vi "PID.vi"(7 "KD":dbl, 8 "Initial feedback in":dbl, 9 "KI":dbl, 10 "Error in":dbl, 11 "KP":dbl) -> (3 "PIDout":dbl)   [LabVIEW 2016]
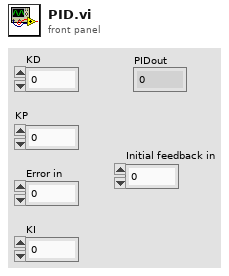
[diagram p1: front panel]
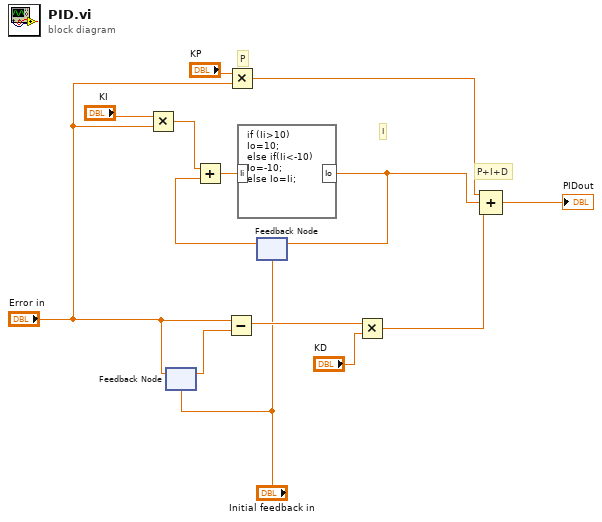
[diagram p0: block diagram]
diagram:
  # "P+I+D"
  # "P"
  # "I"
  n1 = Multiply(x="KI", y="Error in") -> (x*y=w2:dbl)
  n2 = feedback #1("Initial feedback in") -> (w6:dbl)
  n3 = feedback-in #1("Error in") -> ()
  n4 = Subtract(x="Error in", y=w6) -> (x-y=w5:dbl)
  n5 = Multiply(x="KP", y="Error in") -> (x*y=w11:dbl)
  n6 = feedback #2("Initial feedback in") -> (w13:dbl)
  n7 = Add(x=w2, y=w13) -> (x+y=w12:dbl)
  n8 = formula code="if (Ii>10)\nIo=10;\nelse if(Ii<-10)\nIo=-10;\nelse Io=Ii;"("Ii"=w12) -> ("Io"=w3:dbl)
  n9 = feedback-in #2(w3) -> ()
  n10 = Multiply(x=w5, y="KD") -> (x*y=w10:dbl)
  n11 = Compound Arithmetic op=ADD(w11, w3, w10) -> (→"PIDout":dbl)
